vi "TA_Plot.vi"() -> ()   [LabVIEW 2025]
uses:
  TA_DATA.ctl
  <vilib>/Math Plots/3D Math Plots/3D Surface/3D Surface XCtrl/3D Surface.xctl
  <vilib>/Math Plots/3D Math Plots/3D Surface/3D Surface Datatype/Public/Plot Helper (Vector).vi
  <vilib>/Math Plots/3D Math Plots/3D Surface/3D Surface Datatype/3D Surface Datatype.lvclass
panel:
  in  "File Path":path=path "/Users/tm/Desktop/fs-TA/Data/demo_fsta.dat"
  out "TA Data":T1
  in  "Selected\nWavelength":dbl[](array[numeric])
  in  "Selected\nDelay Time":dbl[](array[numeric])
  in  "Update\nSelected\nWavelength":bool
  in  "Apply\nSelected\nDelay Time":bool
  out "TA Selected Kinetics":cluster{"Array":dbl[], "Array 2":dbl[]}[](graph)
  out "TA 3D Surface":refnum<class "3D Plot Datatype.lvclass">[](xcontrol)
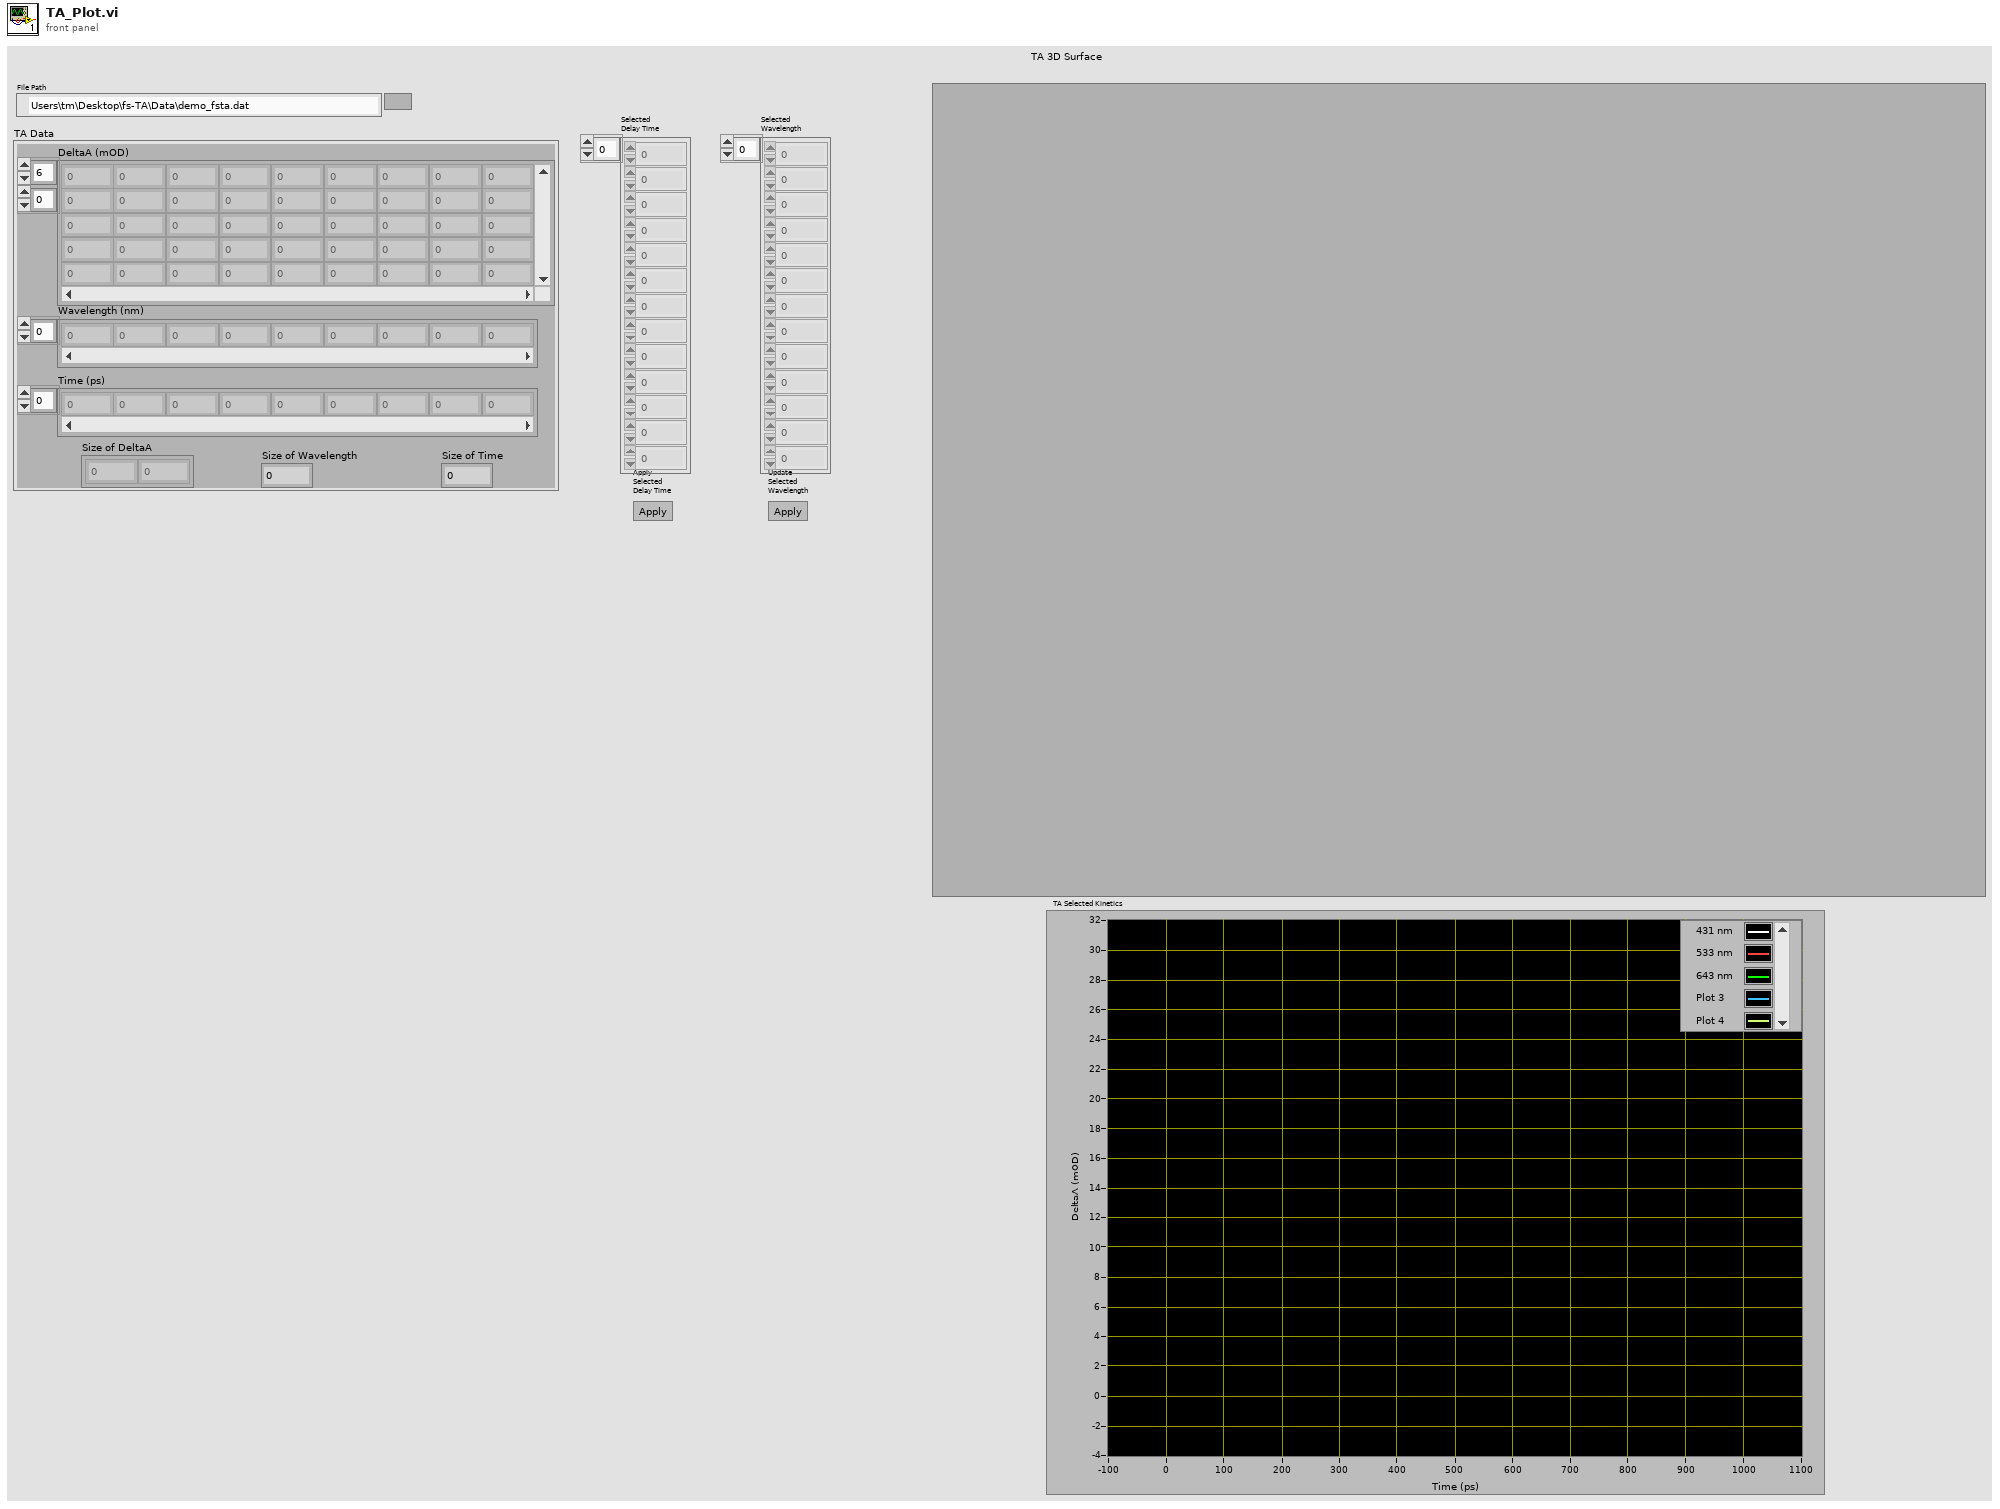
[diagram p1: front panel]
types:
  T1 = typedef "TA_DATA.ctl" = cluster{"DeltaA (mOD)":dbl[][], "Wavelength (nm)":dbl[], "Time (ps)":dbl[], "Size of DeltaA":i32[], "Size of Wavelength":i32, "Size of Time":i32}
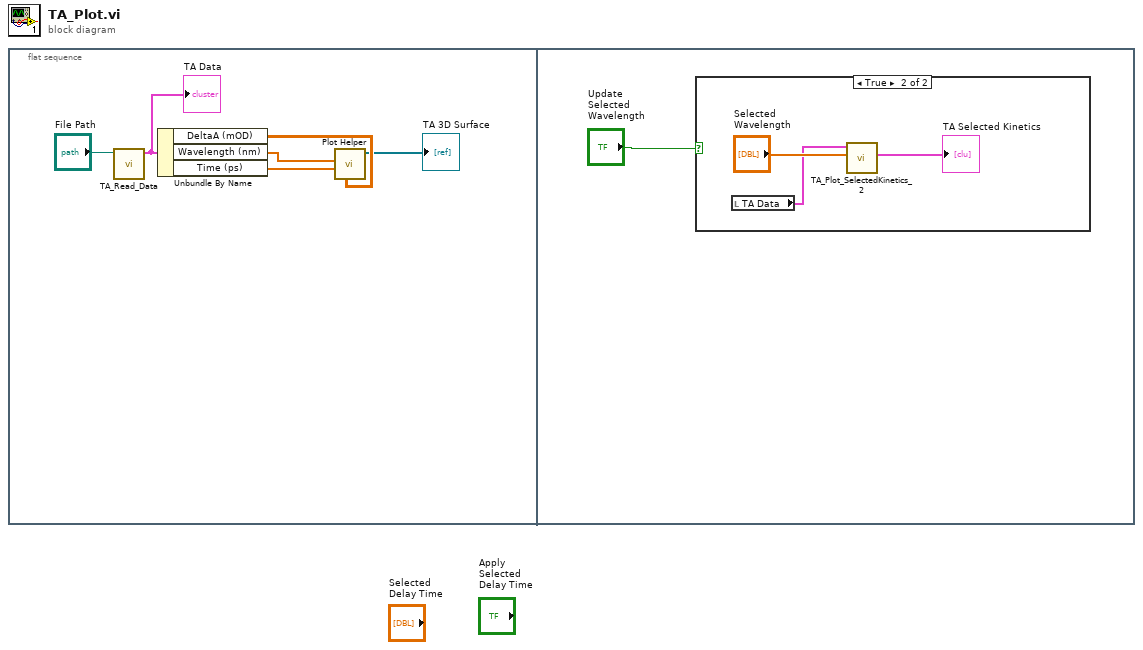
[diagram p0: block diagram]
diagram:
  n1 = flat-sequence {
    frame #0 {
      n2 = call "TA_Read_Data.vi"("File Path"="File Path") -> ("TA Data"=w1:T1)  [unwired: 10 in]
      "TA Data" <- w1
      n3 = Unbundle By Name(w1) -> ("DeltaA (mOD)"=w5:dbl[][], "Wavelength (nm)"=w3:dbl[], "Time (ps)"=w4:dbl[])
      n4 = call-poly <vilib>:"Plot Helper.vi"("z matrix"=w5, "y vector"=w4, "x vector"=w3) -> ("3D Plot lvclass Array out"=→"TA 3D Surface":refnum<class "3D Plot Datatype.lvclass">[])  [unwired: 3 in, 5 out]
    }
    frame #1 {
      n5 = case shown="True" "Update\nSelected\nWavelength" {
        frame False {
        }
        frame True {
          n6 = local read "TA Data"() -> (w8:T1)
          n7 = call "TA_Plot_SelectedKinetics_2.vi"("Selected\nWavelength (nm)"="Selected\nWavelength", "TA Data"=w8) -> ("TA Selected Kinetics"=→"TA Selected Kinetics":cluster{"Array":dbl[], "Array 2":dbl[]}[])  [unwired: 6 in, 1 out]
        }
      }
    }
  }
